vi "Sub_Calculate2DWeights.vi"(2 "Sensor data list":T1=[{"Temperature value"=0.0, "Sensor name"="", "Sensor enabled"=FALSE, "Sensor number in receive list"=0, "Sensor location height"=0, "Sensor location width"=0, "Simulation weight"=[], "Error occured"=FALSE, "Ambient sensor"=FALSE}, {"Temperature value"=0.0, "Sensor name"="", "Sensor enabled"=TRUE, "Sensor number in receive list"=0, "Sensor location height"=0, "Sensor location width"=0, "Simulation weight"=[], "Error occured"=FALSE, "Ambient sensor"=FALSE}, {"Temperature value"=0.0, "Sensor name"="", "Sensor enabled"=TRUE, "Sensor number in receive list"=0, "Sensor location height"=0, "Sensor location width"=0, "Simulation weight"=[], "Error occured"=FALSE, "Ambient sensor"=FALSE}, {"Temperature value"=0.0, "Sensor name"="", "Sensor enabled"=TRUE, "Sensor number in receive list"=0, "Sensor location height"=0, "Sensor location width"=0, "Simulation weight"=[], "Error occured"=FALSE, "Ambient sensor"=FALSE}, {"Temperature value"=0.0, "Sensor name"="", "Sensor enabled"=TRUE, "Sensor number in receive list"=0, "Sensor location height"=0, "Sensor location width"=0, "Simulation weight"=[], "Error occured"=FALSE, "Ambient sensor"=FALSE}, {"Temperature value"=0.0, "Sensor name"="", "Sensor enabled"=TRUE, "Sensor number in receive list"=0, "Sensor location height"=0, "Sensor location width"=0, "Simulation weight"=[], "Error occured"=FALSE, "Ambient sensor"=FALSE}, {"Temperature value"=0.0, "Sensor name"="", "Sensor enabled"=TRUE, "Sensor number in receive list"=0, "Sensor location height"=0, "Sensor location width"=0, "Simulation weight"=[], "Error occured"=FALSE, "Ambient sensor"=FALSE}, {"Temperature value"=0.0, "Sensor name"="", "Sensor enabled"=TRUE, "Sensor number in receive list"=0, "Sensor location height"=0, "Sensor location width"=0, "Simulation weight"=[], "Error occured"=FALSE, "Ambient sensor"=FALSE}, {"Temperature value"=0.0, "Sensor name"="", "Sensor enabled"=TRUE, "Sensor number in receive list"=0, "Sensor location height"=0, "Sensor location width"=0, "Simulation weight"=[], "Error occured"=FALSE, "Ambient sensor"=FALSE}, {"Temperature value"=0.0, "Sensor name"="", "Sensor enabled"=TRUE, "Sensor number in receive list"=0, "Sensor location height"=0, "Sensor location width"=0, "Simulation weight"=[], "Error occured"=FALSE, "Ambient sensor"=FALSE}, {"Temperature value"=0.0, "Sensor name"="", "Sensor enabled"=TRUE, "Sensor number in receive list"=0, "Sensor location height"=0, "Sensor location width"=0, "Simulation weight"=[], "Error occured"=FALSE, "Ambient sensor"=FALSE}, {"Temperature value"=0.0, "Sensor name"="", "Sensor enabled"=TRUE, "Sensor number in receive list"=0, "Sensor location height"=0, "Sensor location width"=0, "Simulation weight"=[], "Error occured"=FALSE, "Ambient sensor"=FALSE}, {"Temperature value"=0.0, "Sensor name"="\n ", "Sensor enabled"=TRUE, "Sensor number in receive list"=0, "Sensor location height"=0, "Sensor location width"=0, "Simulation weight"=[], "Error occured"=FALSE, "Ambient sensor"=FALSE}], 3 "Height scaling":dbl=1.0, 4 "Width scaling":dbl=1.0, 5 "Simulation parameters":cluster{"Object height":u8, "Object width":u8}, 8 "Standard deviation":dbl) -> (6 "Sensor information output":T1)   [LabVIEW 2021]
uses:
  Typedefs/MainApp_SensorData_t.ctl
panel:
  # "Inputs:"
  # "Outputs:"
  # "Required:"
  # "Optional:"
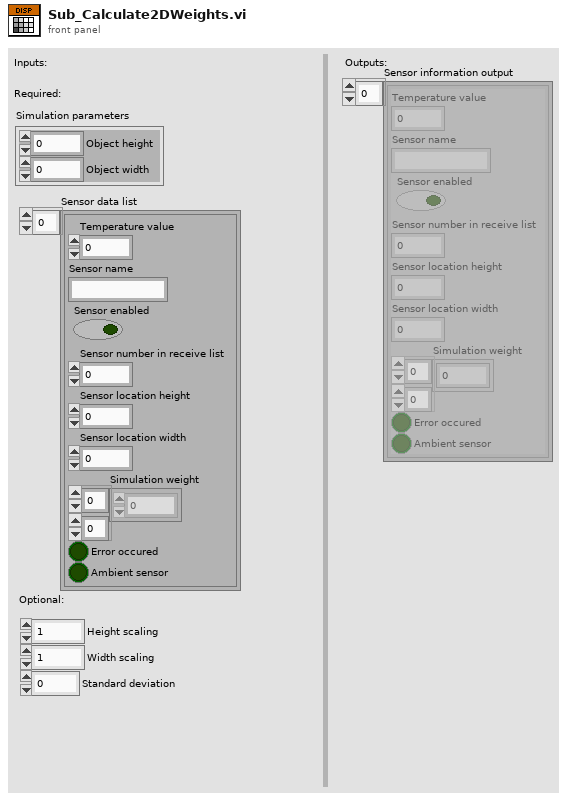
[diagram p1: front panel]
types:
  T1 = typedef "MainApp_SensorData_t.ctl" = cluster{"Temperature value":dbl, "Sensor name":string, "Sensor enabled":bool, "Sensor number in receive list":i32, "Sensor location height":u8, "Sensor location width":u8, "Simulation weight":dbl[][], "Error occured":bool, "Ambient sensor":bool}[]
  T2 = cluster{"Temperature value":dbl, "Sensor name":string, "Sensor enabled":bool, "Sensor number in receive list":i32, "Sensor location height":u8, "Sensor location width":u8, "Simulation weight":dbl[][], "Error occured":bool, "Ambient sensor":bool}
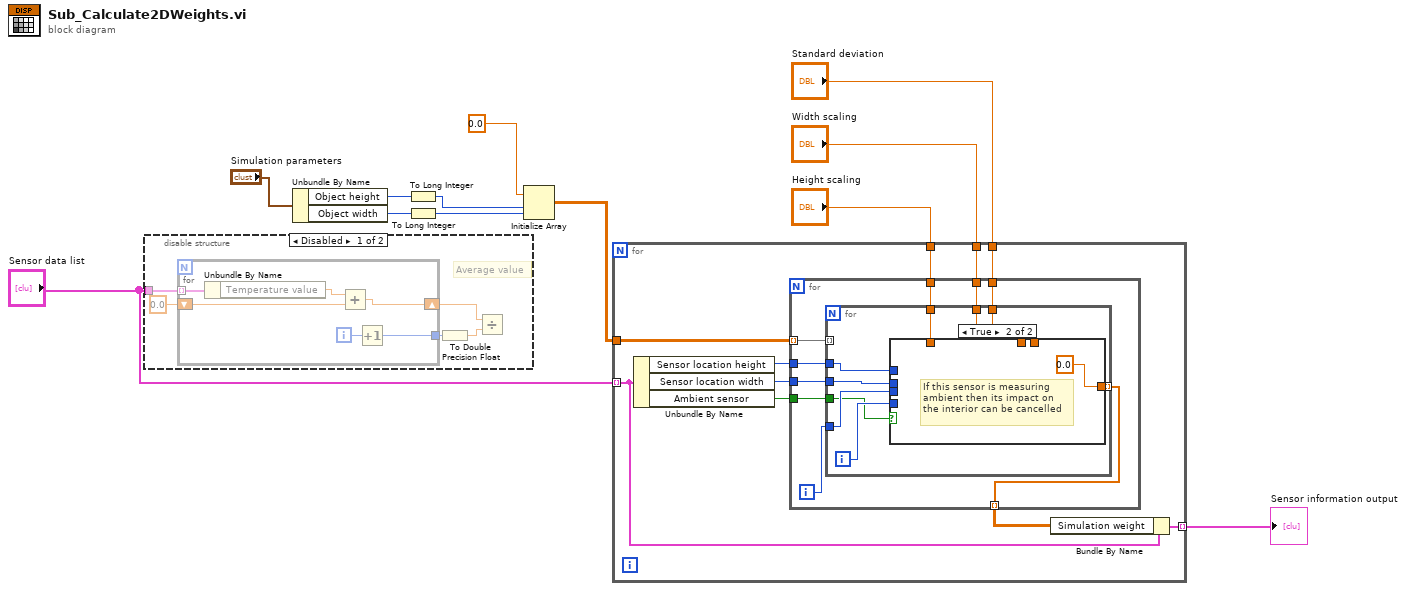
[diagram p0: block diagram]
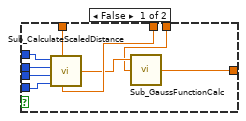
[diagram p3: hidden frame]
diagram:
  n1 = disable-structure shown="Disabled" {
    disable-tunnel: "Sensor data list" -> [w14 _]
    frame Disabled {
      # "Average value"
      n2 = for {
        tunnel: w14 -> [w23] mode=indexing
        shift-right: [w19] -> w15
        shift-left: 0.0 -> [w21]
        tunnel: [w18] -> w16
        i -> [w20]
        n3 = Unbundle By Name(w23) -> ("Temperature value"=w22:dbl)
        n4 = Add(x=w22, y=w21) -> (x+y=w19:dbl)
        n5 = Increment(x=w20) -> (x+1=w18:i32)
      }
      n6 = To Double Precision Float(number=w16) -> (double precision float=w13:dbl)
      n7 = Divide(x=w15, y=w13) -> ()  [unwired: 1 out]
    }
    frame Enabled {
    }
  }
  n8 = Unbundle By Name("Simulation parameters") -> ("Object height"=w9:u8, "Object width"=w11:u8)
  n9 = To Long Integer(number=w9) -> (32bit integer=w5:i32)
  n10 = To Long Integer(number=w11) -> (32bit integer=w4:i32)
  n11 = Initialize Array(0.0 ("element"), w5, w4) -> (w10:dbl[][])
  n12 = for {
    tunnel: "Sensor data list" -> [w27] mode=indexing
    tunnel: "Height scaling" -> [w30]
    tunnel: "Width scaling" -> [w29]
    tunnel: "Standard deviation" -> [w28]
    tunnel: w10 -> [w33]
    tunnel: [w25] -> w1 mode=indexing
    n13 = Unbundle By Name(w27) -> ("Sensor location height"=w32:u8, "Sensor location width"=w31:u8, "Ambient sensor"=w24:bool)
    n14 = for {
      tunnel: w33 -> [w42] mode=indexing
      tunnel: w32 -> [w40]
      tunnel: w31 -> [w39]
      tunnel: w30 -> [w38]
      tunnel: w29 -> [w37]
      tunnel: w28 -> [w36]
      tunnel: [w35] -> w26 mode=indexing
      tunnel: w24 -> [w34]
      i -> [w41]
      n15 = for {
        tunnel: w42 -> [_] mode=indexing
        tunnel: w41 -> [w48]
        tunnel: w40 -> [w51]
        tunnel: w39 -> [w50]
        tunnel: w38 -> [w47]
        tunnel: w37 -> [w46]
        tunnel: w36 -> [w45]
        tunnel: [w44] -> w35 mode=indexing
        tunnel: w34 -> [w43]
        i -> [w49]
        n16 = case shown="True" w43 {
          tunnel: w51 -> [w60 _]
          tunnel: w50 -> [w59 _]
          tunnel: w49 -> [w52 _]
          tunnel: w48 -> [w58 _]
          tunnel: w47 -> [w57 _]
          tunnel: w46 -> [w56 _]
          tunnel: w45 -> [w54 _]
          tunnel: [w53 0.0 ("Gaussian output")] -> w44
          frame False {
            n17 = call "Sub_CalculateScaledDistance.vi"("Width scaling"=w56, "Height scaling"=w57, "Width iteration"=w52, "Height iteration"=w58, "Object width"=w59, "Object height"=w60) -> ("Scaled distance"=w55:dbl)
            n18 = call "Sub_GaussFunctionCalc.vi"("Standard deviation"=w54, "Input"=w55) -> ("Gaussian output"=w53:dbl)  [unwired: 1 in]
          }
          frame True {
            # "If this sensor is measuring\nambient then its impact on\nthe interior can be cancelled"
          }
        }
      }
    }
    n19 = Bundle By Name(cluster=w27, "Simulation weight"=w26) -> (w25:T2)
  }
  "Sensor information output" <- w1
